vi "Read Signal Generator.lvclass.vi"(11 "RF Power in":refnum<class "RF Power.lvclass">) -> (2 "Signal Generator.lvclass":refnum<class "Signal Generator.lvclass">, 3 "RF Power out":refnum<class "RF Power.lvclass">)   [LabVIEW 2020, in "RF Power.lvclass"]
uses:
  RF Power.lvclass
  Instruments/Signal Generator/Signal Generator.lvclass
  RF Power.lvclass/RF Power.ctl
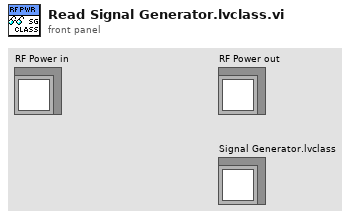
[diagram p1: front panel]
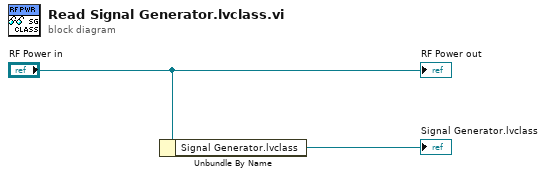
[diagram p0: block diagram]
diagram:
  n1 = Unbundle By Name("RF Power in") -> ("Signal Generator.lvclass"=→"Signal Generator.lvclass":refnum<class "Signal Generator.lvclass">)
  "RF Power out" <- "RF Power in"
